vi "GetGraphTypeInfo.vi"(0 "reference in":refnum<class "StateDiagramGraph.lvclass">, 5 "error in (no error)":errorcluster) -> (14 "reference out":refnum<class "StateDiagramGraph.lvclass">, 15 "GraphTypeName":string, 16 "NodeTypes":refnum<class "AbstractNode.lvclass">[](array[class]), 17 "EdgeTypes":refnum<class "AbstractEdge.lvclass">[](array[class]), 18 "GraphTypeUserName":string, 19 "error out":errorcluster)   [LabVIEW 2016, in "StateDiagramGraph.lvclass"]
uses:
  <resource>/Framework/Providers/Open_GDS/UML/StateDiagramGraph_class/StateDiagramGraph.lvclass
  <resource>/Framework/Providers/Open_GDS/UML/AbstractNode_class/AbstractNode.lvclass
  <resource>/Framework/Providers/Open_GDS/UML/AbstractEdge_class/AbstractEdge.lvclass
  <resource>/Framework/Providers/Open_GDS/UML/NoteNode_class/NoteNode.lvclass
  C:/Program Files (x86)/National Instruments/LabVIEW 2016/resource/Framework/Providers/Open_GDS/UML/AbstractNode_class/AbstractNode.lvclass
  <resource>/Framework/Providers/Open_GDS/UML/NoteEdge_class/NoteEdge.lvclass
  C:/Program Files (x86)/National Instruments/LabVIEW 2016/resource/Framework/Providers/Open_GDS/UML/GeneralPathEdge_class/GeneralPathEdge.lvclass
  <resource>/Framework/Providers/Open_GDS/UML/StateNode_class/StateNode.lvclass
  <resource>/Framework/Providers/Open_GDS/UML/InitialStateNode_class/InitialStateNode.lvclass
  <resource>/Framework/Providers/Open_GDS/UML/FinalStateNode_class/FinalStateNode.lvclass
  <resource>/Framework/Providers/Open_GDS/UML/ChoiceNode_class/ChoiceNode.lvclass
  <resource>/Framework/Providers/Open_GDS/UML/StateTransitionEdge_class/StateTransitionEdge.lvclass
  <resource>/Framework/Providers/Open_GDS/UML/PointNode_class/PointNode.lvclass
  <resource>/Framework/Providers/Open_GDS/UML/GeneralPathEdge_class/GeneralPathEdge.lvclass
  C:/Program Files (x86)/National Instruments/LabVIEW 2016/resource/Framework/Providers/Open_GDS/UML/AbstractEdge_class/AbstractEdge.lvclass
  <resource>/Framework/Providers/Open_GDS/UML/Graph_class/Graph.lvclass
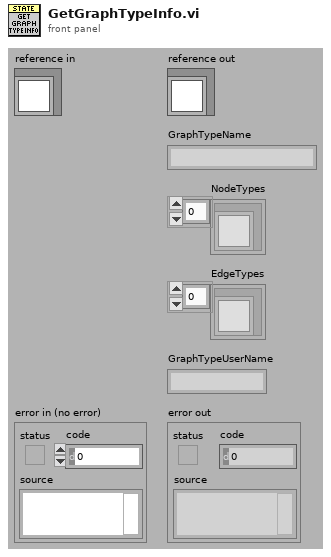
[diagram p1: front panel]
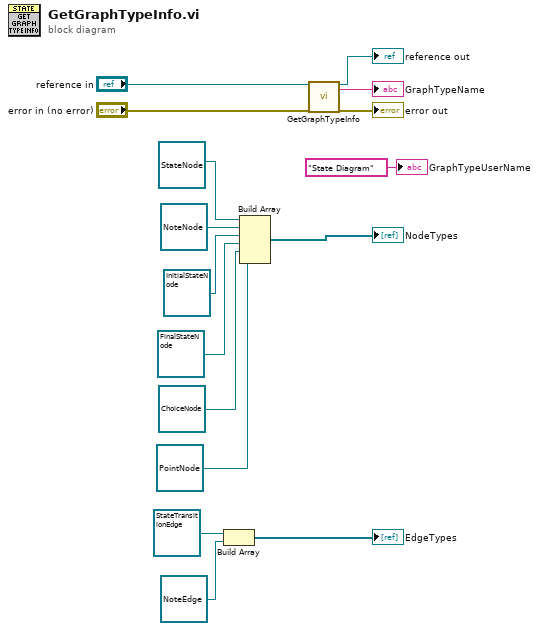
[diagram p0: block diagram]
diagram:
  n1 = Build Array(refnum<class "StateTransitionEdge.lvclass"> refnum ("StateTransitionEdge.lvclass"), refnum<class "NoteEdge.lvclass"> refnum ("NoteEdge.lvclass")) -> (→"EdgeTypes":refnum<class "GeneralPathEdge.lvclass">[])
  n2 = Build Array(refnum<class "StateNode.lvclass"> refnum ("StateNode.lvclass"), refnum<class "NoteNode.lvclass"> refnum ("NoteNode.lvclass"), refnum<class "InitialStateNode.lvclass"> refnum ("InitialStateNode.lvclass"), refnum<class "FinalStateNode.lvclass"> refnum ("FinalStateNode.lvclass"), refnum<class "ChoiceNode.lvclass"> refnum ("ChoiceNode.lvclass"), refnum<class "PointNode.lvclass"> refnum ("PointNode.lvclass")) -> (→"NodeTypes":refnum<class "AbstractNode.lvclass">[])
  n3 = call-parent "GetGraphTypeInfo.vi"("reference in"="reference in", "error in (no error)"="error in (no error)") -> ("reference out"=→"reference out":refnum<class "StateDiagramGraph.lvclass">, "GraphTypeName"=→"GraphTypeName":string, "error out"=→"error out":errorcluster)  [unwired: 12 in, 3 out]
  "GraphTypeUserName" <- "State Diagram" ("GraphTypeUserName")
